vi "[SubVI]FSR_Calculation.vi"(0 "Right FSR Input":dbl, 1 "Left FSR Input":dbl, 2 "Right Input Array":u32[](array[numeric]), 3 "Left Input Array":u32[](array[numeric]), 4 "Elapsed Time":i32) -> (5 "Right Output Array":u32[](array[numeric]), 6 "Left Output Array":u32[](array[numeric]), 7 "Right Cadence Time":dbl format="%0.2f", 8 "Left Cadence Time":dbl format="%0.2f", 9 "Right Gait Phase":dbl, 10 "Left Gait Phase":dbl)   [LabVIEW 2017]
uses:
  <vilib>/Analysis/baseanly.llb/Mean (DBL).vi
  <vilib>/functionblocks/Edge Detection/One Shot Rising with Input/One Shot Rising with Input.vi
  <vilib>/functionblocks/FB Core/FB Core.xnode
  <vilib>/Analysis/NI_AALBase.lvlib
  <vilib>/functionblocks/NI_FunctionBlock Libraries.lvlib
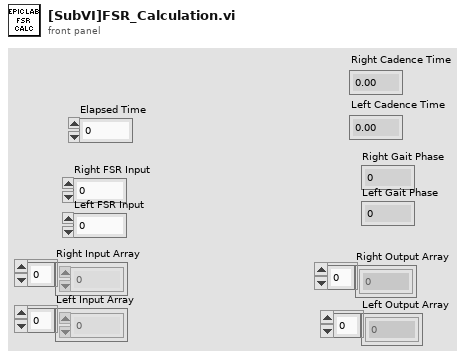
[diagram p1: front panel]
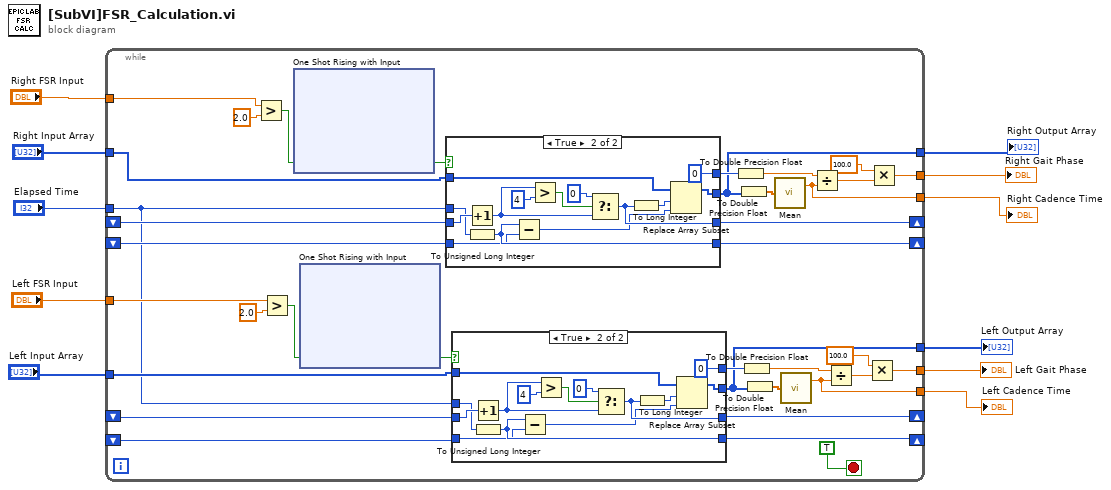
[diagram p0: block diagram]
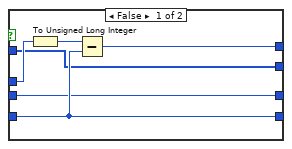
[diagram p2: hidden frame]
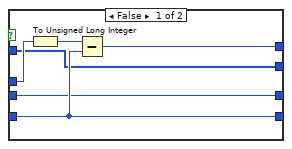
[diagram p3: hidden frame]
diagram:
  n1 = while {
    shift-right: [w38] -> _
    shift-left: _ -> [w36]
    shift-right: [w40] -> _
    shift-left: _ -> [w41]
    tunnel: [w12] -> w11
    tunnel: "Right FSR Input" -> [w34]
    tunnel: "Elapsed Time" -> [w20]
    tunnel: "Right Input Array" -> [w37]
    tunnel: [w35] -> w7
    tunnel: "Left FSR Input" -> [w27]
    tunnel: "Left Input Array" -> [w26]
    tunnel: [w25] -> w4
    shift-right: [w24] -> _
    shift-left: _ -> [w22]
    shift-right: [w23] -> _
    shift-left: _ -> [w21]
    tunnel: [w19] -> w3
    tunnel: [w18] -> w2
    tunnel: [w15] -> w1
    stop <- TRUE ("stop") stop-if-true
    n2 = Greater?(x=w34, y=2.0) -> (0:w46:bool)
    n3 = Greater?(x=w27, y=2.0) -> (0:w32:bool)
    n4 = xnode "One Shot Rising with Input"("input"=w46) -> ("output"=w44:bool)  [unwired: 1 in, 1 out]
    n5 = xnode "One Shot Rising with Input"("input"=w32) -> ("output"=w30:bool)  [unwired: 1 in, 1 out]
    n6 = case shown="True" w44 {
      tunnel: w36 -> [w144 w160]
      tunnel: w20 -> [w148 w158]
      tunnel: [w147 u32 0] -> w42
      tunnel: w41 -> [w146 w156]
      tunnel: [w146 w157] -> w40
      tunnel: w37 -> [w145 w153]
      tunnel: [w145 w150] -> w35
      tunnel: [w144 w155] -> w38
      frame False {
        n7 = To Unsigned Long Integer(number=w148) -> (unsigned 32bit integer=w149:u32)
        n8 = Subtract(x=w149, y=w146) -> (x-y=w147:u32)
      }
      frame True {
        n9 = Increment(x=w160) -> (x+1=w159:u8)
        n10 = To Unsigned Long Integer(number=w158) -> (unsigned 32bit integer=w157:u32)
        n11 = Subtract(x=w157, y=w156) -> (x-y=w151:u32)
        n12 = Greater?(x=w159, y=u8 4) -> (0:w163:bool)
        n13 = Select(t=u8 0, s=w163, f=w159) -> (s? t:f=w155:u8)
        n14 = To Long Integer(number=w155) -> (32bit integer=w152:i32)
        n15 = Replace Array Subset(array=w153, new element=w151, index=w152) -> (w150:u32[])
      }
    }
    n16 = case shown="True" w30 {
      tunnel: w22 -> [w86 w102]
      tunnel: w20 -> [w90 w100]
      tunnel: [w89 u32 0] -> w29
      tunnel: w21 -> [w88 w98]
      tunnel: [w88 w99] -> w23
      tunnel: w26 -> [w87 w95]
      tunnel: [w87 w92] -> w25
      tunnel: [w86 w97] -> w24
      frame False {
        n17 = To Unsigned Long Integer(number=w90) -> (unsigned 32bit integer=w91:u32)
        n18 = Subtract(x=w91, y=w88) -> (x-y=w89:u32)
      }
      frame True {
        n19 = Increment(x=w102) -> (x+1=w101:u8)
        n20 = To Unsigned Long Integer(number=w100) -> (unsigned 32bit integer=w99:u32)
        n21 = Subtract(x=w99, y=w98) -> (x-y=w93:u32)
        n22 = Greater?(x=w101, y=u8 4) -> (0:w105:bool)
        n23 = Select(t=u8 0, s=w105, f=w101) -> (s? t:f=w97:u8)
        n24 = To Long Integer(number=w97) -> (32bit integer=w94:i32)
        n25 = Replace Array Subset(array=w95, new element=w93, index=w94) -> (w92:u32[])
      }
    }
    n26 = To Double Precision Float(number=w42) -> (double precision float=w39:dbl)
    n27 = To Double Precision Float(number=w35) -> (double precision float=w45:dbl[])
    n28 = To Double Precision Float(number=w29) -> (double precision float=w28:dbl)
    n29 = To Double Precision Float(number=w25) -> (double precision float=w31:dbl[])
    n30 = call-poly <vilib>:"Mean.vi"("X"=w45) -> ("mean"=w19:dbl)  [unwired: 1 out]
    n31 = call-poly <vilib>:"Mean.vi"("X"=w31) -> ("mean"=w18:dbl)  [unwired: 1 out]
    n32 = Divide(x=w39, y=w19) -> (x/y=w13:dbl)
    n33 = Divide(x=w28, y=w18) -> (x/y=w17:dbl)
    n34 = Multiply(x=100.0, y=w17) -> (x*y=w15:dbl)
    n35 = Multiply(x=100.0, y=w13) -> (x*y=w12:dbl)
  }
  "Right Gait Phase" <- w11
  "Right Output Array" <- w7
  "Left Gait Phase" <- w1
  "Left Output Array" <- w4
  "Right Cadence Time" <- w3
  "Left Cadence Time" <- w2
